vi "Demo1_Publisher.vi"() -> ()   [LabVIEW 2019]
uses:
  <vilib>/LabVIEW Open Source Project/OpenSerializer/Serializer/Serializer.lvclass
  <vilib>/LabVIEW Open Source Project/MQTT Connection/MQTT_Base/Base Class/MQTT_Base.lvclass/MQTT_Base.ctl
  <vilib>/LabVIEW Open Source Project/MQTT Client/Client class/Client.lvclass/Client.ctl
  <vilib>/LabVIEW Open Source Project/MQTT TCP Connection/MQTT_TCP/Connection/TCPConnection.lvclass
  C:/Program Files (x86)/National Instruments/LabVIEW 2019/vi.lib/LabVIEW Open Source Project/MQTT Connection/MQTT_Connection/Connection/Connection.lvclass
  <vilib>/LabVIEW Open Source Project/MQTT Client/Client class/Client.lvclass
  C:/Program Files (x86)/National Instruments/LabVIEW 2019/vi.lib/LabVIEW Open Source Project/MQTT Connection/MQTT_Base/Base Class/MQTT_Base.lvclass
  <vilib>/LabVIEW Open Source Project/OpenSerializer/Serializer.FlattenedString/Serializer.FlattenedString.lvclass
  C:/Program Files (x86)/National Instruments/LabVIEW 2019/vi.lib/LabVIEW Open Source Project/OpenSerializer/Serializer/Serializer.lvclass
  <vilib>/LabVIEW Open Source Project/MQTT Control Packets/Control Packets/PUBLISH/PUBLISH.lvclass
  <vilib>/LabVIEW Open Source Project/MQTT Connection/MQTT_Base/Base Class/MQTT_Base.lvclass
  <vilib>/LabVIEW Open Source Project/OpenSerializer.Base64/Serializer.Base64.lvclass
  <vilib>/LabVIEW Open Source Project/OpenSerializer JKI JSON/Serializer.JSON.lvclass
panel:
  in  "Connection":bool
  in  "Stop Client":bool
  out "Published":bool
  out "Waveform Chart":dbl(graph)
  out "last error":errorcluster
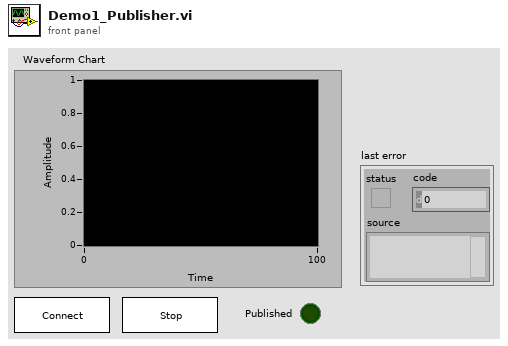
[diagram p1: front panel]
types:
  T1 = typedef "MQTT Client.lvlib/Client.lvclass/Public Events -- cluster.ctl" = cluster{"Connection Status":refnum<user-event>, "Connected":refnum<user-event>, "Application Message":refnum<user-event>}
  T2 = typedef "MQTT Base.lvlib/MQTT_Base.lvclass/Public Events -- cluster.ctl" = cluster{"Stop Event":refnum<user-event>, "Error Event":refnum<user-event>, "Inbound Message":refnum<user-event>}
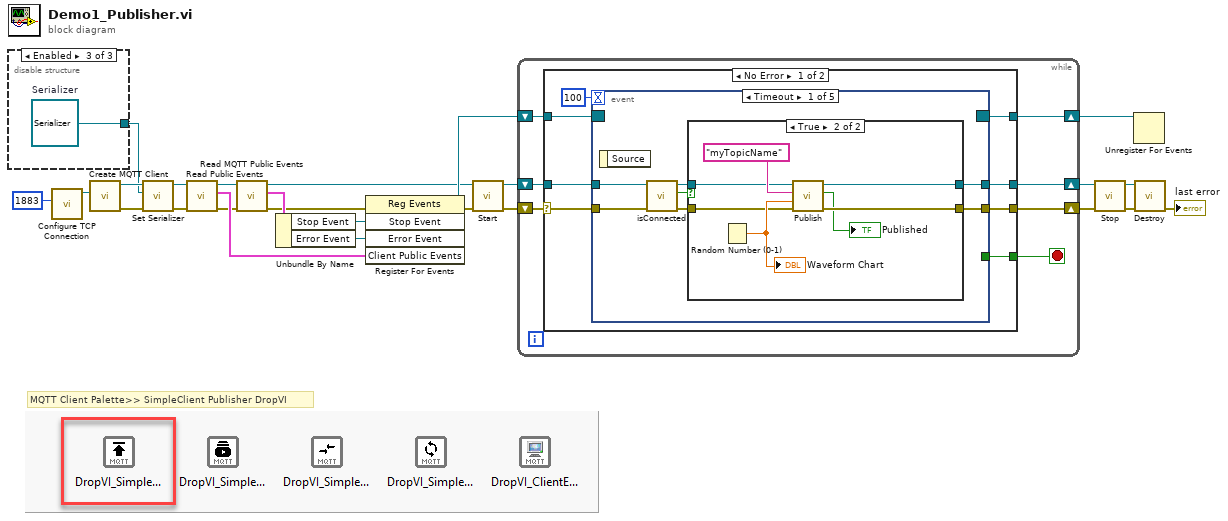
[diagram p0: block diagram]
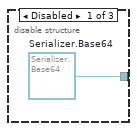
[diagram p2: hidden frame]
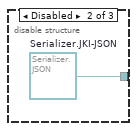
[diagram p3: hidden frame]
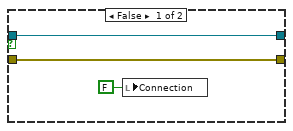
[diagram p4: hidden frame]
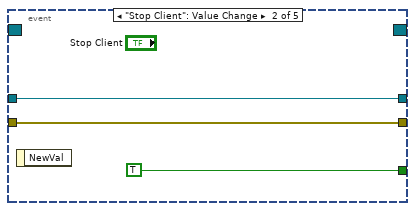
[diagram p5: hidden frame]
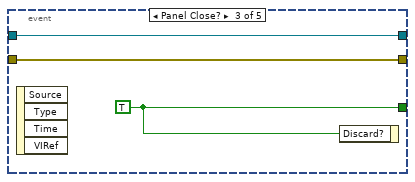
[diagram p6: hidden frame]
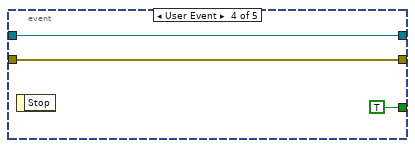
[diagram p7: hidden frame]
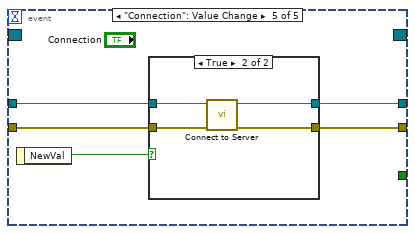
[diagram p8: hidden frame]
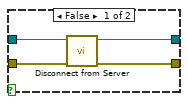
[diagram p9: hidden frame]
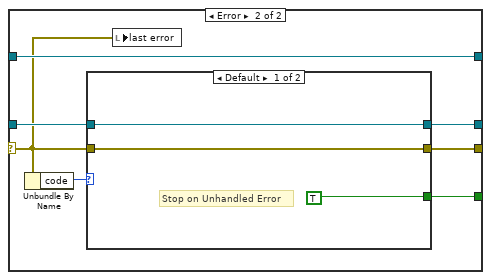
[diagram p10: hidden frame]
diagram:
  # "MQTT Client Palette>> SimpleClient Publisher DropVI"
  n1 = disable-structure shown="Enabled" {
    disable-tunnel: [w26 w27 w28] -> w1
    frame Disabled {
      w26 = refnum<class "Serializer.Base64.lvclass"> refnum  # Serializer.Base64
    }
    frame Disabled {
      w27 = refnum<class "Serializer.JSON.lvclass"> refnum  # Serializer.JKI-JSON
    }
    frame Enabled {
      w28 = refnum<class "Serializer.lvclass"> refnum  # Serializer
    }
  }
  n2 = call <vilib>:"Configure TCP Connection.vi"("remote port (80)"=u16 1883) -> ("TCPConnection"=w6:refnum<class "TCPConnection.lvclass">)  [unwired: 9 in, 1 out]
  n3 = call <vilib>:"Create MQTT Client.vi"("Connection Configuration"=w6) -> ("error out"=w3:errorcluster, "Client out"=w5:refnum<class "Client.lvclass">)  [unwired: 9 in]
  n4 = call <vilib>:"Set Serializer.vi"("error in (no error)"=w3, "Serializer (default: Flattened String)"=w1, "MQTT_Base"=w5) -> ("error out"=w2:errorcluster, "MQTT_Base out"=w4:refnum<class "Client.lvclass">)  [unwired: 7 in]
  n5 = call <vilib>:"Read Public Events.vi"("error in (no error)"=w2, "Client in"=w4) -> ("error out"=w9:errorcluster, "Client Public Events"=w11:T1, "Client out"=w8:refnum<class "Client.lvclass">)  [unwired: 7 in]
  n6 = call <vilib>:"Read MQTT Public Events.vi"("error in (no error)"=w9, "MQTT_Base in"=w8) -> ("error out"=w10:errorcluster, "MQTT Public Events"=w18:T2, "MQTT_Base out"=w13:refnum<class "Client.lvclass">)  [unwired: 7 in]
  n7 = Unbundle By Name(w18) -> ("Stop Event"=w16:refnum<user-event>, "Error Event"=w17:refnum<user-event>)
  n8 = register-events(error in=w10, w16, w17, w11) -> (reference out=w14:refnum<event-registration>, error out=w12:errorcluster)  [unwired: 1 in]
  n9 = call <vilib>:"Start.vi"("error in (no error)"=w12, "MQTT_Base in"=w13) -> ("error out"=w24:errorcluster, "MQTT_Base out"=w23:refnum<class "Client.lvclass">)  [unwired: 7 in, 1 out]
  n10 = while {
    shift-right: [w34] -> w15
    shift-left: w14 -> [w35]
    shift-right: [w31] -> w20
    shift-left: w23 -> [w32]
    shift-right: [w33] -> w22
    shift-left: w24 -> [w29]
    stop <- w30 stop-if-true
    n11 = case shown="No Error" w29 {
      selector: w29 -> [w36 w83]
      tunnel: w35 -> [w43 w89]
      tunnel: [w42 w89] -> w34
      tunnel: [w41 w85] -> w33
      tunnel: w32 -> [w39 w87]
      tunnel: [w38 w86] -> w31
      tunnel: [w37 w84] -> w30
      frame No Error {
        n12 = event shown="[0] Timeout" {
          selector: w43 -> [_ _ _ _ _]
          dyn-events: [_ _ _ _ _] -> w42
          timeout: 100 -> [_ _ _ _ _]
          tunnel: w36 -> [w46 w62 w64 w69 w70]
          tunnel: [w49 w62 w64 w69 w71] -> w41
          tunnel: [_ TRUE w66 TRUE _] -> w37
          tunnel: w39 -> [w48 w63 w65 w67 w74]
          tunnel: [w50 w63 w65 w67 w72] -> w38
          event Timeout {
            n13 = event-data() -> ()  [unwired: 1 in, 1 out]
            n14 = call <vilib>:"isConnected.vi"("error in (no error)"=w46, "Client in"=w48) -> ("error out"=w45:errorcluster, "connected"=w44:bool, "Client out"=w47:refnum<class "Client.lvclass">)  [unwired: 7 in]
            n15 = case shown="True" w44 {
              tunnel: [w53 w59] -> w50
              tunnel: [w52 w58] -> w49
              tunnel: w47 -> [w53 w55]
              tunnel: w45 -> [w52 w54]
              frame False {
                n16 = local write "Connection"(FALSE ("Connection")) -> ()
              }
              frame True {
                n17 = Random Number (0-1)() -> (number: 0 to 1=w56:dbl)
                "Waveform Chart" <- w56
                n18 = call <vilib>:"Publish.vi"("error in (no error)"=w54, "Payload"=w56, "Topic Name (empty: Payload name)"="myTopicName", "Client in"=w55) -> ("error out"=w58:errorcluster, "Published"=→"Published":bool, "Client out"=w59:refnum<class "Client.lvclass">)  [unwired: 5 in]
              }
            }
          }
          event "Stop Client": Value Change {
            n19 = event-data() -> ()  [unwired: 1 in, 1 out]
          }
          event Panel Close? {
            w66 = TRUE
            n20 = event-data() -> ()  [unwired: 1 in, 4 out]
            n21 = event-data("Discard?"=w66) -> ()  [unwired: 1 in, 1 out]
          }
          event User Event {
            n22 = event-data() -> ()  [unwired: 1 in, 1 out]
          }
          event "Connection": Value Change {
            n23 = event-data() -> ("NewVal"=w73:bool)  [unwired: 1 in]
            n24 = case shown="True" w73 {
              tunnel: w74 -> [w78 w82]
              tunnel: [w77 w79] -> w72
              tunnel: [w76 w80] -> w71
              tunnel: w70 -> [w75 w81]
              frame False {
                n25 = call <vilib>:"Disconnect from Server.vi"("error in (no error)"=w75, "Client in"=w78) -> ("error out"=w76:errorcluster, "Client out"=w77:refnum<class "Client.lvclass">)  [unwired: 7 in, 1 out]
              }
              frame True {
                n26 = call <vilib>:"Connect to Server.vi"("error in (no error)"=w81, "Client in"=w82) -> ("error out"=w80:errorcluster, "Client out"=w79:refnum<class "Client.lvclass">)  [unwired: 6 in, 2 out]
              }
            }
          }
        }
      }
      frame Error {
        n27 = Unbundle By Name(w83) -> ("code"=w88:i32)
        n28 = case shown="Default" w88 {
          tunnel: w87 -> [w92 w93]
          tunnel: [w92 w93] -> w86
          tunnel: w83 -> [w91 _]
          tunnel: [w91 _] -> w85
          tunnel: [TRUE _] -> w84
          frame Default {
            # "Stop on Unhandled Error"
          }
          frame 56, 63, 66 {
            # "Disconnected"
          }
        }
        n29 = local write "last error"(w83) -> ()
      }
    }
  }
  n30 = call <vilib>:"Stop.vi"("error in (no error)"=w22, "MQTT_Base in"=w20) -> ("error out"=w21:errorcluster, "MQTT_Base out"=w19:refnum<class "Client.lvclass">)  [unwired: 7 in, 1 out]
  n31 = Unregister For Events(event registration refnum=w15) -> ()  [unwired: 1 in, 1 out]
  n32 = call <vilib>:"Destroy.vi"("error in (no error)"=w21, "MQTT_Base in"=w19) -> ("error out"=→"last error":errorcluster)  [unwired: 8 in, 1 out]
